vi "Binary Search 1D Array.vi"(10 "element":dbl, 11 "1D array sorted":dbl[](array[numeric])) -> (1 "Path Complete?":bool, 2 "index":i32, 3 "value":dbl)   [LabVIEW 2019]
panel:
  in  "offset (0)":i32
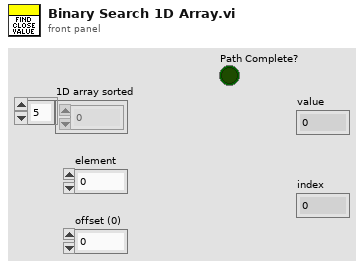
[diagram p1: front panel]
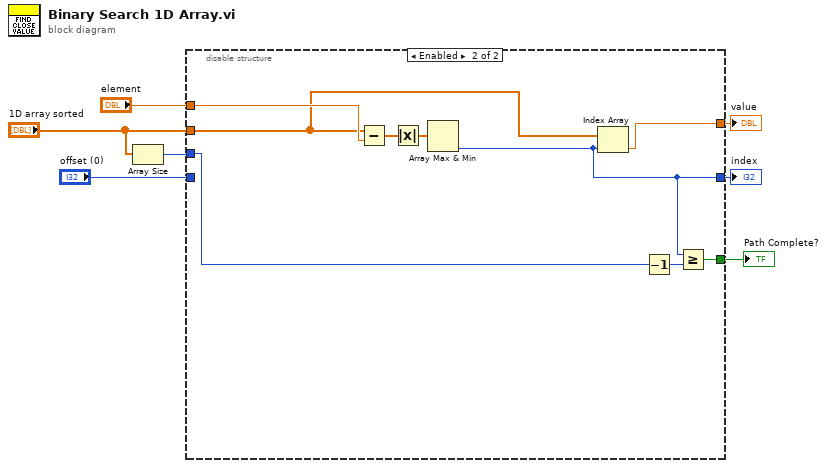
[diagram p0: block diagram]
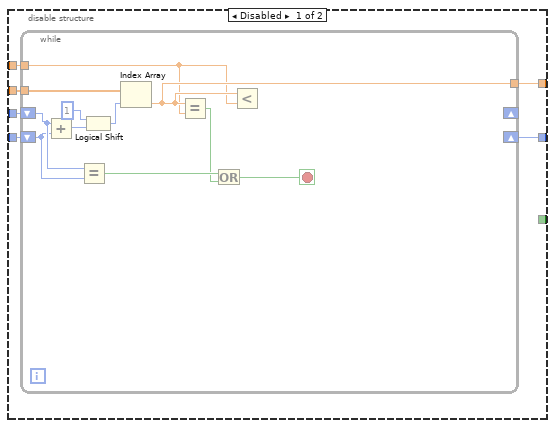
[diagram p2: hidden frame]
diagram:
  n1 = Array Size(array="1D array sorted") -> (size(s)=w5:i32)
  n2 = disable-structure shown="Enabled" {
    disable-tunnel: [w13 w29] -> w7
    disable-tunnel: "offset (0)" -> [w12 _]
    disable-tunnel: w5 -> [w11 w27]
    disable-tunnel: "1D array sorted" -> [w10 w30]
    disable-tunnel: "element" -> [w9 w33]
    disable-tunnel: [w8 w28] -> w2
    disable-tunnel: [_ w25] -> w1
    frame Disabled {
      n3 = while {
        tunnel: w10 -> [w22]
        tunnel: w9 -> [w14]
        shift-right: _ -> [_]
        shift-left: w11 -> [w20]
        shift-right: [_] -> w8
        shift-left: w12 -> [w19]
        tunnel: [w15] -> w13
        stop <- w16 stop-if-true
        n4 = Add(x=w20, y=w19) -> (x+y=w24:i32)
        n5 = Equal?(x=w20, y=w19) -> (x = y?=w18:bool)
        n6 = Logical Shift(y=i16 1, x=w24) -> (x << y=w21:i32)
        n7 = Index Array(array=w22, index=w21) -> (element=w15:dbl)
        n8 = Equal?(x=w15, y=w14) -> (x = y?=w17:bool)
        n9 = Or(x=w18, y=w17) -> (x .or. y?=w16:bool)
        n10 = Less?(x=w15, y=w14) -> ()  [unwired: 1 out]
      }
    }
    frame Enabled {
      n11 = Subtract(x=w30, y=w33) -> (x-y=w32:dbl[])
      n12 = Absolute Value(x=w32) -> (abs(x)=w31:dbl[])
      n13 = Array Max & Min(array=w31) -> (min index (indices)=w28:i32)  [unwired: 3 out]
      n14 = Index Array(array=w30, index=w28) -> (element=w29:dbl)
      n15 = Decrement(x=w27) -> (x-1=w26:i32)
      n16 = Greater Or Equal?(x=w28, y=w26) -> (x >= y?=w25:bool)
    }
  }
  "value" <- w7
  "index" <- w2
  "Path Complete?" <- w1
